vi "Halt.vi"(6 "balls":T1[](array[typedef]), 9 "Field Size in":T2, 10 "Numeric":i32, 11 "Robot in":T3) -> (3 "Robot out":T3)   [LabVIEW 2016]
uses:
  Core/AI Robot.ctl
  Functions Enum.ctl
  Core/Field Size.ctl
  Core/AI Ball.ctl
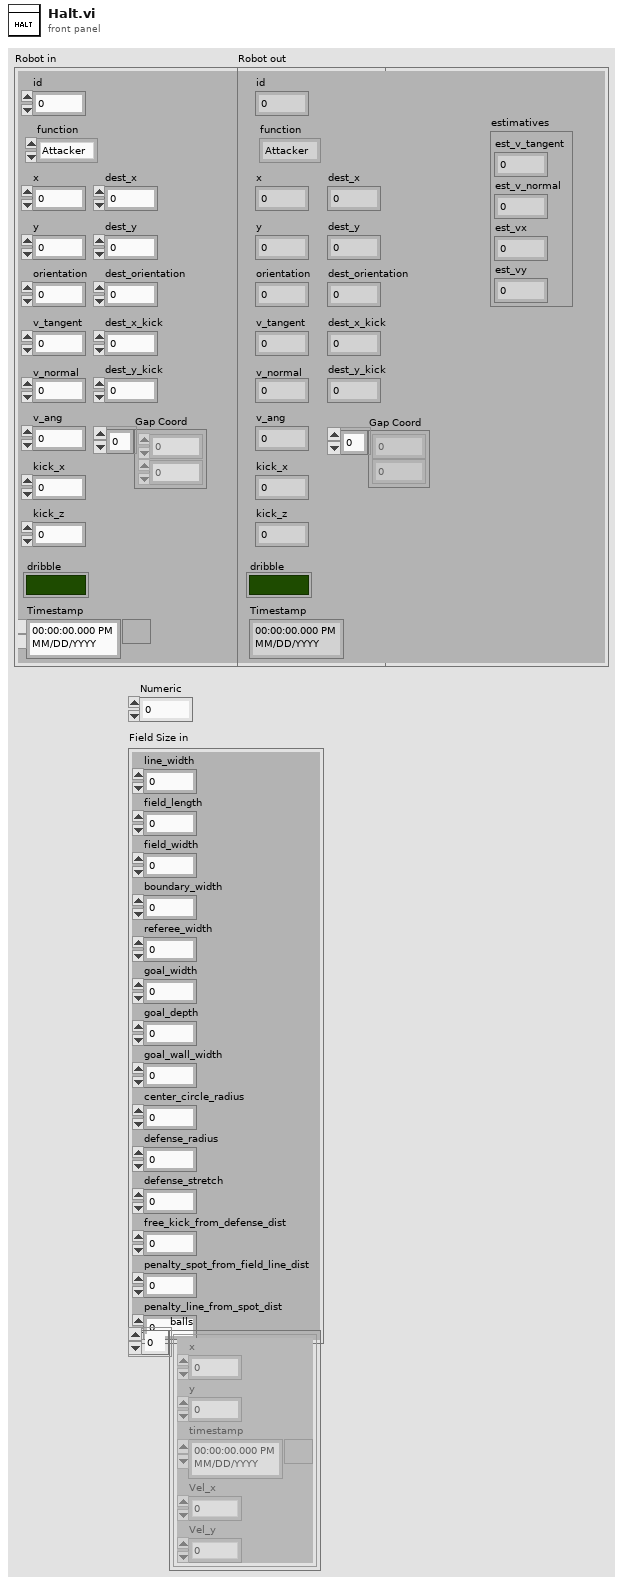
[diagram p1: front panel]
types:
  T1 = typedef "AI Ball.ctl" = cluster{"x":dbl, "y":dbl, "timestamp":timestamp, "Vel_x":dbl, "Vel_y":dbl}
  T2 = typedef "Field Size.ctl" = cluster{"line_width":u32, "field_length":u32, "field_width":u32, "boundary_width":u32, "referee_width":u32, "goal_width":u32, "goal_depth":u32, "goal_wall_width":u32, "center_circle_radius":u32, "defense_radius":u32, "defense_stretch":u32, "free_kick_from_defense_dist":u32, "penalty_spot_from_field_line_dist":u32, "penalty_line_from_spot_dist":u32}
  T3 = typedef "AI Robot.ctl" = cluster{"id":u32, "function":T4, "x":dbl, "y":dbl, "orientation":dbl, "v_tangent":dbl, "v_normal":dbl, "v_ang":dbl, "kick_x":dbl, "kick_z":dbl, "dribble":bool, "Timestamp":timestamp, "dest_x":dbl, "dest_y":dbl, "dest_orientation":dbl, "estimatives":cluster{"est_v_tangent":dbl, "est_v_normal":dbl, "est_vx":dbl, "est_vy":dbl}, "dest_x_kick":dbl, "dest_y_kick":dbl, "Gap Coord":dbl[]}
  T4 = typedef "Functions Enum.ctl" = enum16{"Attacker", "Goalie", "Defender", "Striker", "Goto 0", "Dummy", "Kicker", "ZigZag"}
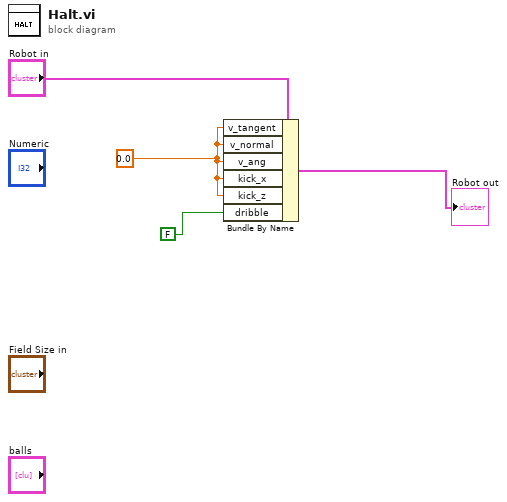
[diagram p0: block diagram]
diagram:
  w2 = 0.0 ("v_normal")
  n1 = Bundle By Name(cluster="Robot in", "v_tangent"=w2, "v_normal"=w2, "v_ang"=w2, "kick_x"=w2, "kick_z"=w2, "dribble"=FALSE) -> (→"Robot out":T3)
